vi "PH_AxisGUI_NF2.ProcEvents.vi"(0 "i ref in":refnum<vi>, 5 "error in":errorcluster) -> (14 "i ref out":refnum<vi>, 19 "error out":errorcluster)   [LabVIEW 2014, in "PH_AxisGUI_NF2.lvlib"]
doc: "This method is used to define the events the object will listen to. Add your own events here."
uses:
  PH_AxisGUI_NF2.lvlib
  CS_Core/BaseProcess/BaseProcess.event definition.ctl
  CS_Core/CAEObj/CAEObj.event definition.ctl
  CS_Core/BaseProcess/BaseProcess.descriptor string definition.ctl
  CS_Core/BaseProcess/BaseProcess.lvlib
  PH_Basics/PH_Common/PH_Common.lvlib
  CS_Core/CAEObj/CAEObj.lvlib
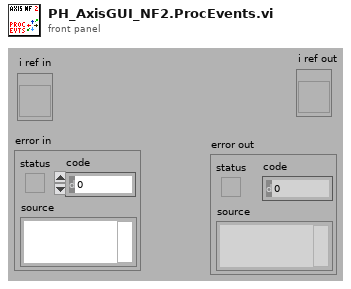
[diagram p1: front panel]
types:
  T1 = typedef "BaseProcess.lvlib/BaseProcess.event definition.ctl" = cluster{"CAEEvtDef":T2, "Data Descriptor":T3}
  T2 = typedef "CAEObj.lvlib/CAEObj.event definition.ctl" = cluster{"URL":string, "enable":bool, "ignoreResID":bool}
  T3 = typedef "BaseProcess.lvlib/BaseProcess.descriptor string definition.ctl" = string
  T4 = typedef "PH_AxisGUI_NF2.lvlib/PH_AxisGUI_NF2.i attribute.ctl" = cluster{"GUI Refs":cluster{"Delete":refnum<vi>, "Instance Status":refnum<vi>, "Width Axis 1":refnum<vi>, "Width Axis 2":refnum<vi>}, "Instance":string, "System":string, "Width Axis 1":i32, "Width Axis 2":i32, "Sign Change Axis 1":bool, "Sign Change Axis 2":bool, "Motor Axis 1":i32, "Motor Axis 2":i32}
  T5 = typedef "PH_Common.lvlib/PH_DIM.Event Declarer.ctl" = cluster{"Service Name":string, "Selector":string}
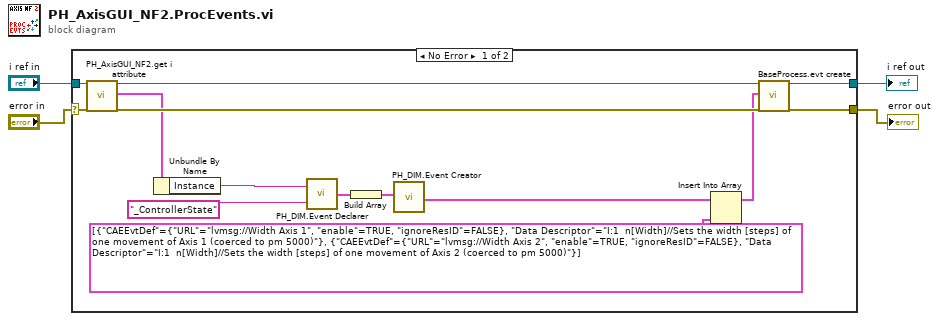
[diagram p0: block diagram]
diagram:
  n1 = case shown="No Error" "error in" {
    selector: "error in" -> [w14 w19]
    tunnel: "i ref in" -> [w16 w20]
    tunnel: [w18 w20] -> w3
    tunnel: [w17 w19] -> w2
    frame No Error {
      n2 = call "PH_AxisGUI_NF2.get i attribute.vi"("i ref in"=w16, "error in (no error)"=w14) -> ("i ref out"=w15:refnum<vi>, "i attribute"=w12:T4, "error out"=w13:errorcluster)  [unwired: 15 in]
      n3 = Unbundle By Name(w12) -> ("Instance"=w7:string)
      n4 = call "PH_DIM.Event Declarer.vi"("Selector"="_ControllerState" ("URL"), "Service Name"=w7) -> ("declared DIM Event"=w5:T5)
      n5 = Build Array(w5) -> (w10:T5[])
      n6 = call "PH_DIM.Event Creator.vi"("Status Services"=w10) -> ("DIM Service Events"=w11:T1[])  [unwired: 18 in]
      n7 = Insert Into Array(array=w11, new element=T1[] [{"CAEEvtDef"={"URL"="lvmsg://Width Axis 1", "enable"=TRUE, "ignoreResID"=FALSE}, "Data Descriptor"="I:1  n[Width]//Sets the width [steps] of one movement of Axis 1 (coerced to pm 5000)"}, {"CAEEvtDef"={"URL"="lvmsg://Width Axis 2", "enable"=TRUE, "ignoreResID"=FALSE}, "Data Descriptor"="I:1  n[Width]//Sets the width [steps] of one movement of Axis 2 (coerced to pm 5000)"}]) -> (w9:T1[])  [unwired: 1 in]
      n8 = call "BaseProcess.evt create.vi"("i ref in"=w15, "newEvents"=w9, "error in (no error)"=w13) -> ("i ref out"=w18:refnum<vi>, "error out"=w17:errorcluster)  [unwired: 13 in, 2 out]
    }
    frame Error {
    }
  }
  "i ref out" <- w3
  "error out" <- w2
